vi "WRP Start Acquisition.vi"(8 "error in (no error)":errorcluster) -> (0 "error out":errorcluster, 3 "function return":i32)   [LabVIEW 2018, in "SesWrapper.lvlib"]
doc: "int STDCALL WRP_StartAcquisition();"
uses:
  SesWrapper.lvlib
  build/Debug/SESWrapper.dll
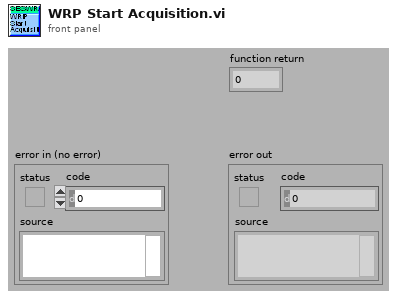
[diagram p1: front panel]
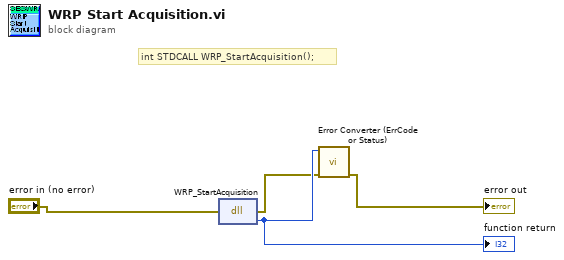
[diagram p0: block diagram]
diagram:
  # "int STDCALL WRP_StartAcquisition();"
  n1 = dll-call lib="C:/Development/svn/seswrapper-lib/build/Debug/SESWrapper.*" fn="WRP_StartAcquisition"(error in="error in (no error)") -> (error out=w2:errorcluster, w4:i32)  [unwired: 2 in, 1 out]
  "function return" <- w4
  n2 = call "Error Converter (ErrCode or Status).vi"("error in (no error)"=w2, "error code"=w4) -> ("error out"=→"error out":errorcluster)  [unwired: 9 in]
